vi "Run.vi"(8 "error in (no error)":errorcluster, 9 "Type of Hexaboard":T1, 10 "Control In":T2={"I-O.lvclass"=refnum, "Gantry"=refnum, "Dispenser"="COM1"}, 11 "Assembly In":refnum<class "Assembly Run.lvclass">) -> (0 "error out":errorcluster, 2 "Control Out":T2={"I-O.lvclass"=refnum, "Gantry"=refnum, "Dispenser"="COM1"}, 3 "Assembly Out":refnum<class "Assembly Run.lvclass">)   [LabVIEW 2021, in "Assembly Run.lvclass"]
uses:
  Assembly Run.lvclass
  Controller/Controllers.ctl
  Controller/I-O/I-O.lvclass
  C:/Program Files (x86)/Aerotech/A3200/LabVIEW/2010/Bin/Aerotech.A3200.dll
  Program Files (x86)/Aerotech/A3200/LabVIEW/2010/Bin/Aerotech.A3200.dll
  Routine/TypeOfHexaboard.ctl
  Assembly Run.lvclass/Assembly Run.ctl
  Workspace/Fixture.lvclass
  Routine/Routine.lvclass
  Controller/Motion/Motion.lvclass
  Controller/Controller.lvclass
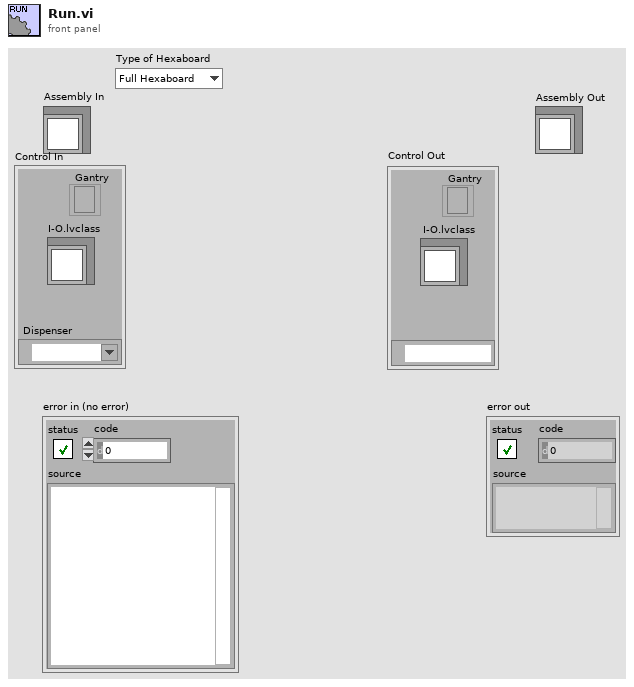
[diagram p1: front panel]
types:
  T1 = typedef "Routine.lvclass/TypeOfHexaboard.ctl" = enum16{"Full Hexaboard", "Right Partial PCB", "Right Partial Sensor", "Al Dummy Right Partial Sensor"}
  T2 = typedef "Controller.lvclass/Controllers.ctl" = cluster{"I-O.lvclass":refnum<class "I-O.lvclass">, "Gantry":refnum<k24>, "Dispenser":refnum<visa-resource-name>}
  T3 = typedef "Fixture.lvclass/Workspace.ctl" = cluster{"XYZTheta":dbl[], "Workspace Valve":i32, "Workspace Sensor":i32}
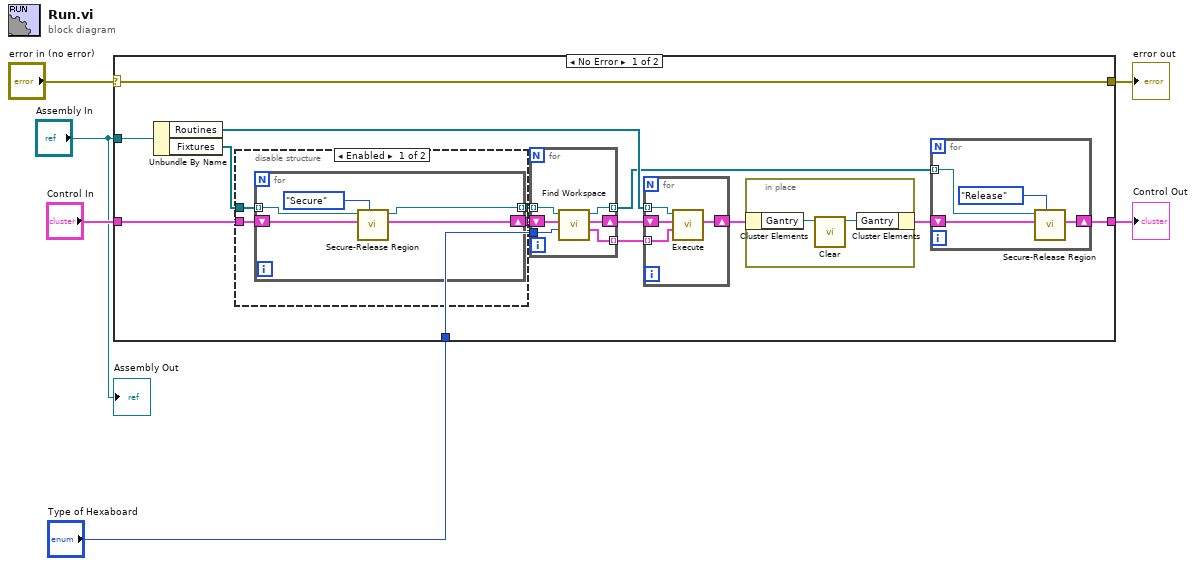
[diagram p0: block diagram]
diagram:
  n1 = case shown="No Error" "error in (no error)" {
    selector: "error in (no error)" -> [w20 w49]
    tunnel: [w20 w49] -> w5
    tunnel: [w14 w48] -> w4
    tunnel: "Assembly In" -> [w12 _]
    tunnel: "Control In" -> [w9 w48]
    tunnel: "Type of Hexaboard" -> [w7 _]
    frame No Error {
      n2 = Unbundle By Name(w12) -> ("Routines"=w19:refnum<class "Routine.lvclass">[], "Fixtures"=w13:refnum<class "Fixture.lvclass">[])
      n3 = disable-structure shown="Enabled" {
        disable-tunnel: [w24 w31] -> w17
        disable-tunnel: w13 -> [w23 w31]
        disable-tunnel: w9 -> [w22 w30]
        disable-tunnel: [w21 w30] -> w8
        frame Enabled {
          n4 = for {
            tunnel: [w29] -> w24 mode=indexing
            tunnel: w23 -> [w28] mode=indexing
            shift-right: [w26] -> w21
            shift-left: w22 -> [w27]
            n5 = call-dynamic "Secure-Release Region.vi"("Action"=enum16{"Secure", "Release"}."Secure", "Control In"=w27, "Fixture in"=w28) -> ("Control Out"=w26:T2, "Fixture out"=w29:refnum<class "Fixture.lvclass">)  [unwired: 6 in, 1 out]
          }
        }
        frame Disabled {
        }
      }
      n6 = for {
        tunnel: w17 -> [w47] mode=indexing
        tunnel: [w45] -> w18 mode=indexing
        tunnel: [w46] -> w16 mode=indexing
        shift-right: [w43] -> w11
        shift-left: w8 -> [w44]
        tunnel: w7 -> [w42]
        n7 = call-dynamic "Find Workspace.vi"("Type of Hexaboard"=w42, "Control In"=w44, "Workspace In"=w47) -> (1:"Workspace Out"=w45:T3, "Control Out"=w43:T2, 3:"Workspace Out"=w46:refnum<class "Fixture.lvclass">)  [unwired: 5 in, 1 out]
      }
      n8 = for {
        tunnel: w19 -> [w41] mode=indexing
        tunnel: w18 -> [w40] mode=indexing
        shift-right: [w38] -> w10
        shift-left: w11 -> [w39]
        n9 = call-dynamic "Execute.vi"("Workspace"=w40, "Control In"=w39, "Routine in"=w41) -> ("Control Out"=w38:T2)  [unwired: 6 in, 2 out]
      }
      n10 = in-place {
        n11 = in-place-cluster #1(w10) -> ("Gantry"=w36:refnum<k24>)
        n12 = call "Clear.vi"("Gantry In"=w36) -> ("Gantry Out"=w37:refnum<k24>)  [unwired: 9 in, 1 out]
        n13 = in-place-cluster #1("Gantry"=w37) -> (w15:T2)
      }
      n14 = for {
        tunnel: w16 -> [w35] mode=indexing
        shift-right: [w34] -> w14
        shift-left: w15 -> [w33]
        n15 = call-dynamic "Secure-Release Region.vi"("Action"=enum16{"Secure", "Release"}."Release", "Control In"=w33, "Fixture in"=w35) -> ("Control Out"=w34:T2)  [unwired: 6 in, 2 out]
      }
    }
    frame Error {
    }
  }
  "error out" <- w5
  "Control Out" <- w4
  "Assembly Out" <- "Assembly In"
